vi "EntryFinshCheck.vi"(9 "file path (dialog if empty)":path, 10 "CurrentEntry":string, 11 "EventProgressDataInput":string[][](array[string])) -> (2 "EventProgress":sgl, 3 "EventProgressDataOut":string[][](array[string]))   [LabVIEW 2013]
uses:
  <vilib>/Utility/file.llb/Read Delimited Spreadsheet (string).vi
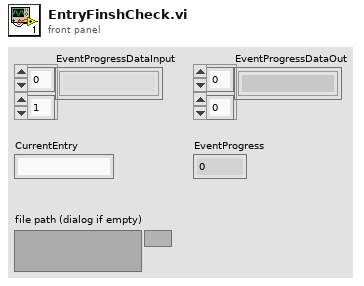
[diagram p1: front panel]
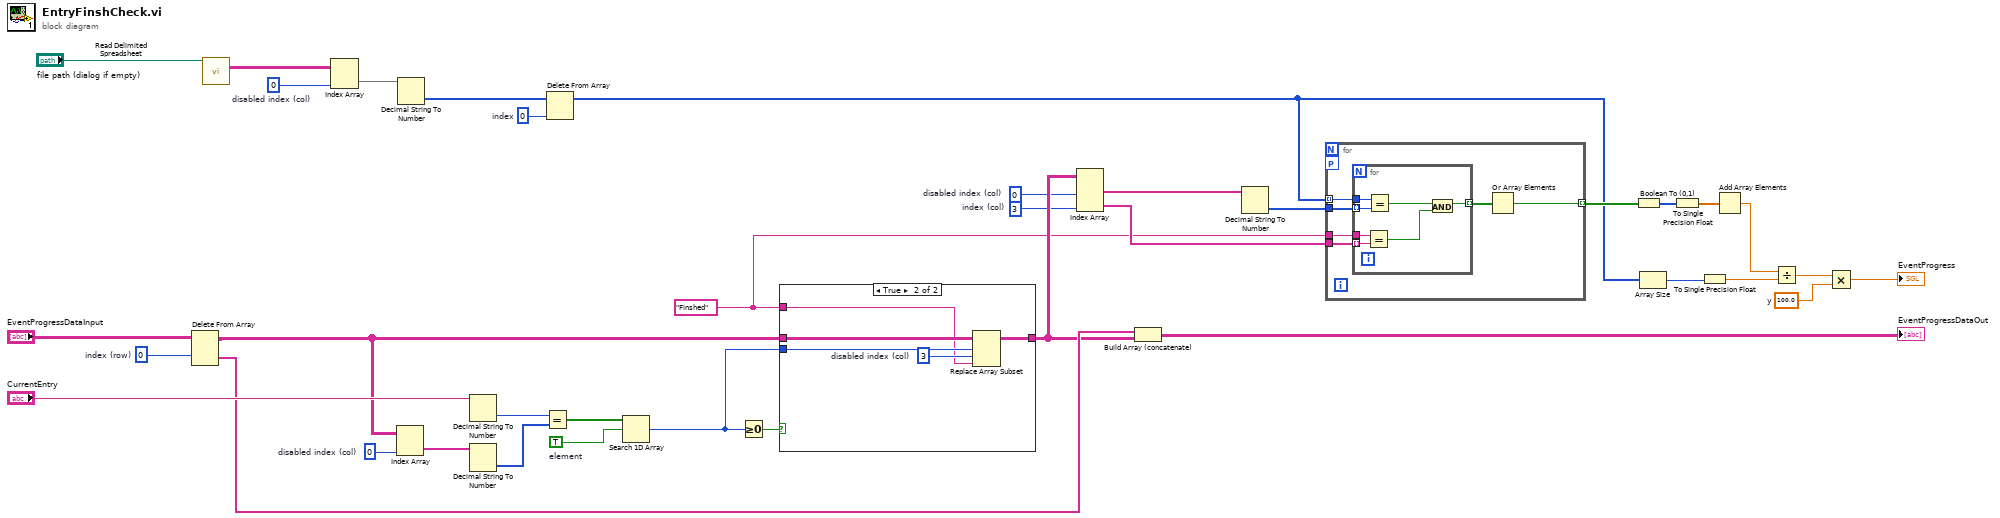
[diagram p0: block diagram]
diagram:
  w2 = "Finshed"
  w4 = 3  # index (col)
  w6 = 0  # index
  w12 = 0  # disabled index (col)
  w15 = 0  # disabled index (col)
  w20 = 0  # index (row)
  w22 = sgl 100.0  # y
  w31 = 0  # disabled index (col)
  w37 = TRUE  # element
  n1 = Delete From Array "Delete From Array"(array="EventProgressDataInput", index (row)=w20) -> (deleted portion=w17:string[], array with subset deleted=w19:string[][])  [unwired: 2 in]
  n2 = call-poly <vilib>:"Read Delimited Spreadsheet.vi"("file path (dialog if empty)"="file path (dialog if empty)") -> ("all rows"=w1:string[][])  [unwired: 9 in, 5 out]
  n3 = Index Array "Index Array"(array=w1, index (col)=w15) -> (element=w14:string[])  [unwired: 1 in]
  n4 = Index Array "Index Array"(array=w19, index (col)=w31) -> (element=w32:string[])  [unwired: 1 in]
  n5 = Decimal String To Number(string=w14) -> (number=w8:i32[])  [unwired: 2 in, 1 out]
  n6 = Decimal String To Number(string="CurrentEntry") -> (number=w35:i32)  [unwired: 2 in, 1 out]
  n7 = Decimal String To Number(string=w32) -> (number=w33:i32[])  [unwired: 2 in, 1 out]
  n8 = Equal?(x=w35, y=w33) -> (x = y?=w36:bool[])
  n9 = Delete From Array "Delete From Array"(array=w8, index=w6) -> (array with subset deleted=w5:i32[])  [unwired: 1 in, 1 out]
  n10 = Search 1D Array(1D array=w36, element=w37) -> (index of element=w29:i32)  [unwired: 1 in]
  n11 = Greater Or Equal To 0?(x=w29) -> (x >= 0?=w30:bool)
  n12 = case shown="True" w30 {
    tunnel: [w38 w43] -> w13
    tunnel: w19 -> [w38 w42]
    tunnel: w29 -> [_ w41]
    tunnel: w2 -> [_ w39]
    frame False {
    }
    frame True {
      w40 = 3  # disabled index (col)
      n13 = Replace Array Subset "Replace Array Subset"(array=w42, new element=w39, index (row)=w41, index (col)=w40) -> (w43:string[][])
    }
  }
  n14 = Index Array "Index Array"(array=w13, index (col) #1=w12, index (col) #2=w4) -> (element #1=w11:string[], element #2=w3:string[])  [unwired: 2 in]
  n15 = Build Array (concatenate) "Build Array"(w17, w13) -> (→"EventProgressDataOut":string[][])
  n16 = Decimal String To Number(string=w11) -> (number=w9:i32[])  [unwired: 2 in, 1 out]
  n17 = for {
    tunnel: w9 -> [w49]
    tunnel: w5 -> [w48] mode=indexing
    workers-P: _ -> [_]
    tunnel: [w46] -> w7 mode=indexing
    tunnel: w3 -> [w45]
    tunnel: w2 -> [w44]
    n18 = for {
      tunnel: w49 -> [w56] mode=indexing
      tunnel: w48 -> [w55]
      tunnel: [w51] -> w47 mode=indexing
      tunnel: w45 -> [w53] mode=indexing
      tunnel: w44 -> [w52]
      n19 = Equal?(x=w52, y=w53) -> (x = y?=w50:bool)
      n20 = Equal?(x=w55, y=w56) -> (x = y?=w54:bool)
      n21 = And(x=w54, y=w50) -> (x .and. y?=w51:bool)
    }
    n22 = Or Array Elements(Boolean array=w47) -> (logical OR=w46:bool)
  }
  n23 = Boolean To (0,1)(Boolean=w7) -> (0, 1=w25:i16[])
  n24 = Array Size(array=w5) -> (size(s)=w23:i32)
  n25 = To Single Precision Float(number=w25) -> (single precision float=w10:sgl[])
  n26 = To Single Precision Float(number=w23) -> (single precision float=w27:sgl)
  n27 = Add Array Elements(numeric array=w10) -> (sum=w24:sgl)
  n28 = Divide(x=w24, y=w27) -> (x/y=w28:sgl)
  n29 = Multiply(x=w28, y=w22) -> (x*y=→"EventProgress":sgl)
